vi "Configure Number of Points.vi"(8 "error in (no error)":errorcluster, 10 "Number of Point":i32, 11 "VNA-ZNB in":refnum<class "VNA-ZNB.lvclass">) -> (0 "error out":errorcluster, 3 "VNA-ZNB out":refnum<class "VNA-ZNB.lvclass">)   [LabVIEW 2020, in "VNA-ZNB.lvclass"]
doc: "Configures the number of points in the sweep.\nThe number of points will be choosen to the nearest supported."
uses:
  VNA-ZNB.lvclass
  C:/Sandbox/RF Bench/Source Code/WiSpry Test Framework/Instruments/Instrument.lvclass
  C:/Sandbox/RF Bench/Source Code/WiSpry Test Framework/Instruments/Vector Network Analyzer/Vector Network Analyzer.lvclass
  Instrument.lvclass/Instrument.ctl
  Vector Network Analyzer.lvclass/Vector Network Analyzer.ctl
  Instrument.lvclass
  Vector Network Analyzer.lvclass
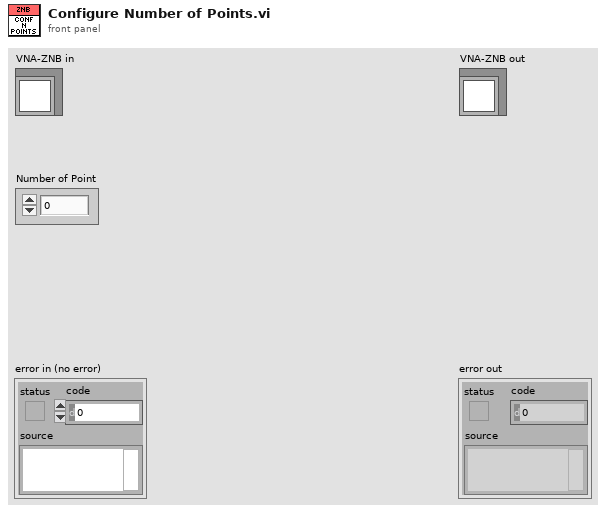
[diagram p1: front panel]
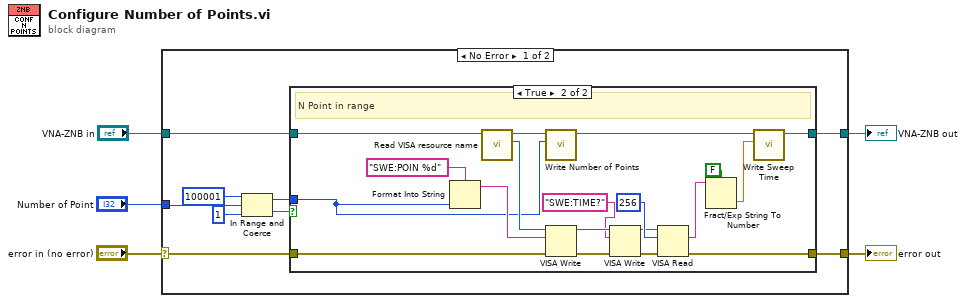
[diagram p0: block diagram]
diagram:
  n1 = case shown="No Error" "error in (no error)" {
    selector: "error in (no error)" -> [w8 w36]
    tunnel: "VNA-ZNB in" -> [w9 w37]
    tunnel: "Number of Point" -> [w14 _]
    tunnel: [w7 w37] -> w1
    tunnel: [w6 w36] -> w2
    frame No Error {
      n2 = In Range and Coerce(upper limit=100001, x=w14, lower limit=1) -> (coerced(x)=w10:i32, In Range?=w11:bool)
      n3 = case shown="True" w11 {
        tunnel: w10 -> [_ w29]
        tunnel: w9 -> [w16 w35]
        tunnel: w8 -> [w15 w31]
        tunnel: [w16 w26] -> w7
        tunnel: [w15 w22] -> w6
        frame False {
          # "Add Error handler"
          # "Raise Error"
        }
        frame True {
          # "N Point in range"
          n4 = Format Into String(format string="SWE:POIN %d", w29) -> (resulting string=w33:string)  [unwired: 2 in, 1 out]
          n5 = call "Read VISA resource name.vi"("Instrument in"=w35) -> ("VISA resource name"=w32:refnum<visa-resource-name>, "Instrument out"=w30:refnum<class "VNA-ZNB.lvclass">)  [unwired: 9 in]
          n6 = call "Write Number of Points.vi"("Number of Points"=w29, "Vector Network Analyzer in"=w30) -> ("Vector Network Analyzer out"=w27:refnum<class "VNA-ZNB.lvclass">)  [unwired: 9 in]
          n7 = VISA Write(VISA resource name=w32, write buffer=w33, error in (no error)=w31) -> (VISA resource name out=w18:refnum<visa-resource-name>, error out=w19:errorcluster)  [unwired: 1 out]
          n8 = VISA Write(VISA resource name=w18, write buffer="SWE:TIME?", error in (no error)=w19) -> (VISA resource name out=w20:refnum<visa-resource-name>, error out=w21:errorcluster)  [unwired: 1 out]
          n9 = VISA Read(VISA resource name=w20, byte count=u32 256, error in (no error)=w21) -> (read buffer=w25:string, error out=w22:errorcluster)  [unwired: 2 out]
          n10 = Fract/Exp String To Number(use system decimal point (T)=FALSE, string=w25) -> (number=w23:dbl)  [unwired: 2 in, 1 out]
          n11 = call "Write Sweep Time.vi"("Sweep Time"=w23, "Vector Network Analyzer in"=w27) -> ("Vector Network Analyzer out"=w26:refnum<class "VNA-ZNB.lvclass">)  [unwired: 9 in]
        }
      }
    }
    frame Error {
    }
  }
  "error out" <- w2
  "VNA-ZNB out" <- w1
